vi "Get date time info.vi"(8 "error in (no error)":errorcluster) -> (0 "error out":errorcluster, 1 "seconds":string, 2 "minutes":string, 3 "hour":string, 4 "time string":string, 5 "date string":string, 6 "AM or PM":string)   [LabVIEW 2013]
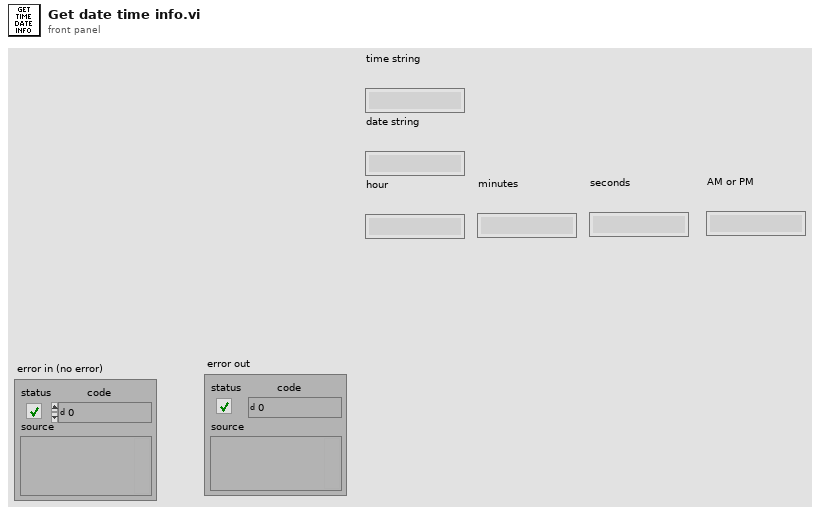
[diagram p1: front panel]
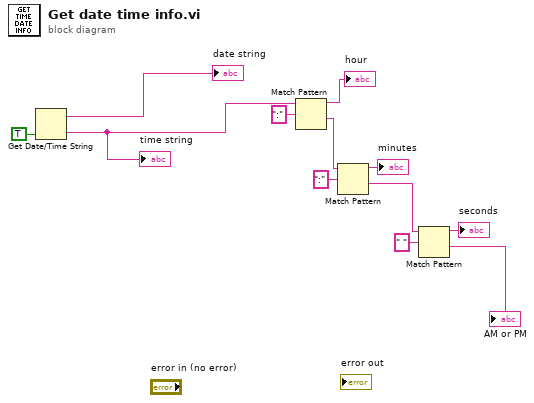
[diagram p0: block diagram]
diagram:
  n1 = Get Date/Time String(want seconds? (F)=TRUE) -> (date string=→"date string":string, time string=w9:string)  [unwired: 2 in]
  "time string" <- w9
  n2 = Match Pattern(string=w9, regular expression=":") -> (before substring=→"hour":string, after substring=w6:string)  [unwired: 1 in, 2 out]
  n3 = Match Pattern(string=w6, regular expression=":") -> (before substring=→"minutes":string, after substring=w3:string)  [unwired: 1 in, 2 out]
  n4 = Match Pattern(string=w3, regular expression=" ") -> (before substring=→"seconds":string, after substring=→"AM or PM":string)  [unwired: 1 in, 2 out]
